vi "Freeform C-Scan Demo.vi"() -> ()   [LabVIEW 2017]
uses:
  Program Files/Thorlabs/SpectralRadar/LabVIEW/2012/user.lib/SpectralRadar.llb/OCT Device.lvclass
  Program Files/Thorlabs/SpectralRadar/LabVIEW/2012/user.lib/SpectralRadar.llb/Probe.lvclass
  Program Files/Thorlabs/SpectralRadar/LabVIEW/2012/user.lib/SpectralRadar.llb/Scan Pattern.lvclass
  Program Files/Thorlabs/SpectralRadar/LabVIEW/2012/user.lib/SpectralRadar.llb/Raw Data Export Format Selection.ctl
panel:
  in  "deltaVY":sgl=0.001
  in  "deltaVX":sgl=0.001
  out "Current B":i32
  out "Time cost":dbl
  out "End time":timestamp
  out "Start time":timestamp
  in  "# Bscan":i32=400
  in  "ARpt":i32=100
  in  "#Ascan":i32=400
  in  "Raw Data Export Format":T1
  in  "Path":path=path "D:/OCT Imaging/EXPERIMENT DATA"
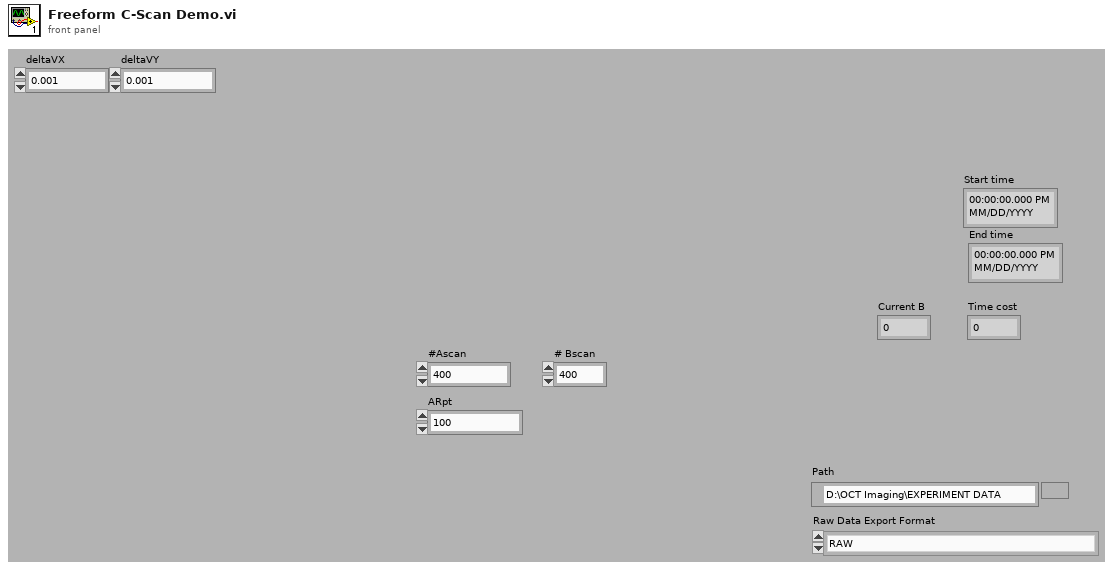
[diagram p1: front panel]
types:
  T1 = typedef "Raw Data Export Format Selection.ctl" = enum16{"RAW", "SRR (Spectral Radar Raw)"}
  T2 = enum16{"Asynchronous Continuous", "Asynchronous Finite", "Synchronous"}
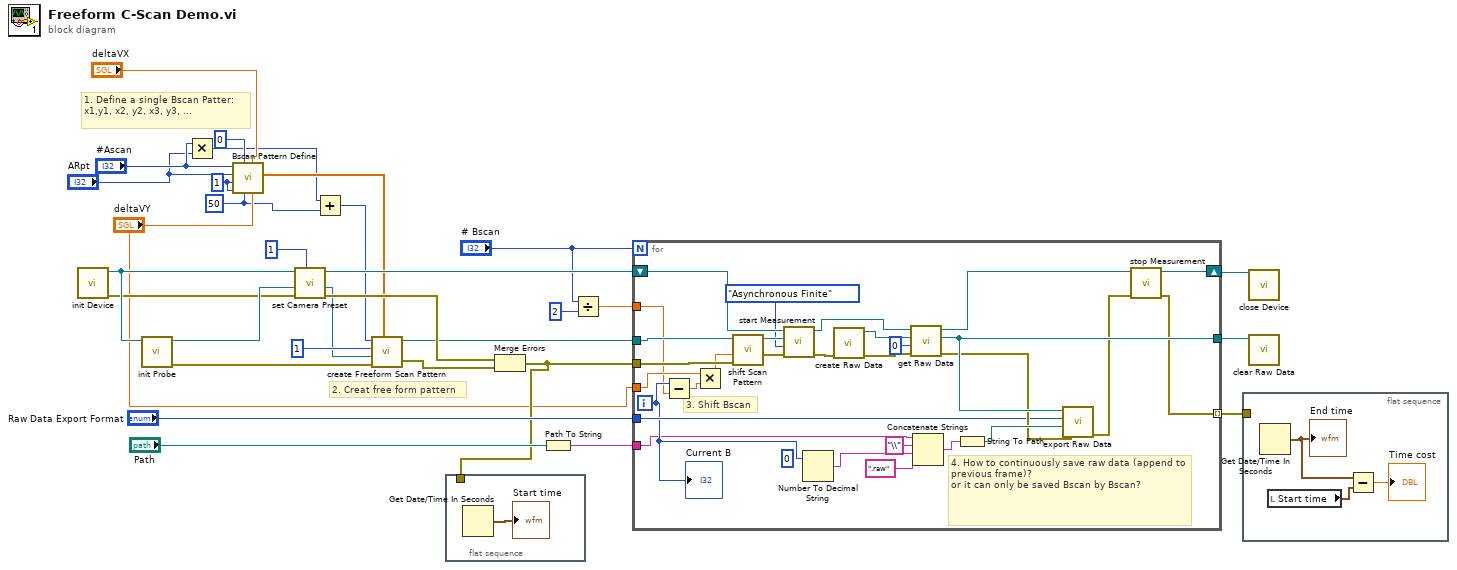
[diagram p0: block diagram]
diagram:
  w4 = 1 ("#Bscan")
  w2 = 50 ("#Brtn_extra")
  # "2. Creat free form pattern"
  # "1. Define a single Bscan Patter: x1,y1, x2, y2, x3, y3, ..."
  n1 = call "init Device.vi"() -> ("error out"=w15:errorcluster, "OCTDevice"=w16:refnum<class "OCT Device.lvclass">)  [unwired: 6 in]
  n2 = call "init Probe.vi"("OCT Device"=w16) -> ("error out"=w17:errorcluster, "GalvoControl"=w29:refnum<class "Probe.lvclass">)  [unwired: 5 in]
  n3 = Multiply(x="#Ascan", y="ARpt") -> (x*y=w3:i32)
  n4 = call "Bscan Pattern Define.vi"("deltaVY"="deltaVY", "deltaVX"="deltaVX", "#Brtn_extra"=w2, "# ARpt_extra"=0, "BRpt"=w4, "#Bscan"=w4, "#ARpt"="ARpt", "#Ascan"="#Ascan") -> ("Scan patter"=w23:dbl[])  [unwired: 2 in, 1 out]
  n5 = call "set Camera Preset.vi"("Numeric"=1, "error in (no error)"=w15, "Probe"=w29, "OCTDevice"=w16) -> ("error out"=w24:errorcluster, "Probe 2"=w20:refnum<class "Probe.lvclass">, "OCTDevice out"=w28:refnum<class "OCT Device.lvclass">)  [unwired: 2 in, 1 out]
  n6 = Add(x=w3, y=w2) -> (x+y=w1:i32)
  n7 = call "create Freeform Scan Pattern.vi"("positions"=w23, "error in (no error)"=w17, "Probe"=w20, "SizeY"=u32 1, "SizeX"=w1) -> ("error out"=w18:errorcluster, "Scan Pattern"=w19:refnum<class "Scan Pattern.lvclass">)  [unwired: 1 in]
  n8 = flat-sequence {
    tunnel: w13 -> [_]
    frame #0 {
      n9 = Get Date/Time In Seconds() -> (seconds since 1Jan1904=→"Start time":timestamp)
    }
  }
  n10 = Merge Errors(w24, w18) -> (w13:errorcluster)
  n11 = Path To String(path="Path") -> (string=w26:string)
  n12 = Divide(x="# Bscan", y=2) -> (x/y=w9:dbl)
  n13 = for {
    N: "# Bscan" -> [_]
    tunnel: w13 -> [w47]
    tunnel: [w58] -> w31
    tunnel: w26 -> [w34]
    tunnel: w19 -> [w48]
    shift-right: [w56] -> w30
    shift-left: w28 -> [w54]
    tunnel: "deltaVY" -> [w43]
    tunnel: "Raw Data Export Format" -> [w41]
    tunnel: [w38] -> w12 mode=indexing
    tunnel: w9 -> [w36]
    i -> [w37]
    (unwired) 0 ("number")
    # "4. How to continuously save raw data (append to previous frame)?\nor it can only be saved Bscan by Bscan?"
    # "3. Shift Bscan"
    n14 = Subtract(x=w37, y=w36) -> (x-y=w35:dbl)
    n15 = Multiply(x=w43, y=w35) -> (x*y=w42:dbl)
    n16 = call "shift Scan Pattern.vi"("error in (no error)"=w47, "Shift Y"=w42, "Scan Pattern in"=w48) -> ("error out"=w46:errorcluster, "Scan Pattern out"=w45:refnum<class "Scan Pattern.lvclass">)  [unwired: 3 in]
    n17 = call "start Measurement.vi"("error in (no error)"=w46, "Acquisition Type"=T2."Asynchronous Finite", "Scan Pattern"=w45, "OCTDevice"=w54) -> ("error out"=w60:errorcluster, "OCTDevice"=w55:refnum<class "OCT Device.lvclass">)  [unwired: 1 in, 1 out]
    n18 = Number To Decimal String(number=w37) -> (decimal integer string=w39:string)  [unwired: 1 in]
    n19 = call "create Raw Data.vi"("error in (no error)"=w60) -> ("error out"=w59:errorcluster, "Raw Data"=w61:refnum<class "Raw Data.lvclass">)  [unwired: 5 in]
    n20 = call "get Raw Data.vi"("error in (no error)"=w59, "Camera Index"=0, "RawData in"=w61, "OCTDevice in"=w55) -> ("error out"=w49:errorcluster, "RawData out"=w58:refnum<class "Raw Data.lvclass">, "OCTDevice out"=w57:refnum<class "OCT Device.lvclass">)  [unwired: 1 in]
    n21 = Concatenate Strings(w34, "\\" ("string"), w39, ".raw" ("string")) -> (w50:string)
    n22 = String To Path(string=w50) -> (path=w51:path)
    n23 = call "export Raw Data.vi"("error in (no error)"=w49, "Export File"=w51, "Raw Data Export Format Selection"=w41, "Data in"=w58) -> ("error out"=w53:errorcluster)  [unwired: 2 in, 1 out]
    n24 = call "stop Measurement.vi"("error in (no error)"=w53, "OCTDevice"=w57) -> ("error out"=w38:errorcluster, "OCTDevice"=w56:refnum<class "OCT Device.lvclass">)  [unwired: 4 in]
    "Current B" <- w37
  }
  n25 = flat-sequence {
    tunnel: w12 -> [_]
    frame #0 {
      n26 = Get Date/Time In Seconds() -> (seconds since 1Jan1904=w64:timestamp)
      "End time" <- w64
      n27 = local read "Start time"() -> (w63:timestamp)
      n28 = Subtract(x=w64, y=w63) -> (x-y=→"Time cost":dbl)
    }
  }
  n29 = call "close Device.vi"("OCTDevice"=w30) -> ()  [unwired: 6 in, 1 out]
  n30 = call "clear Raw Data.vi"("Raw Data"=w31) -> ()  [unwired: 6 in, 1 out]
